vi "SetParam.vi"(7 "RS":bool, 8 "error in (no error)":errorcluster, 9 "Param to Set in":u16, 10 "Visa":refnum<visa-resource-name>) -> (0 "error out":errorcluster)   [LabVIEW 2017]
uses:
  <vilib>/Utility/miscctls.llb/LVMinMaxIncTypeDef.ctl
panel:
  out "RS Out":string
  out "Horizontal Progress Bar":i32(slide) min=0 max=50 scale=0.0..50.0
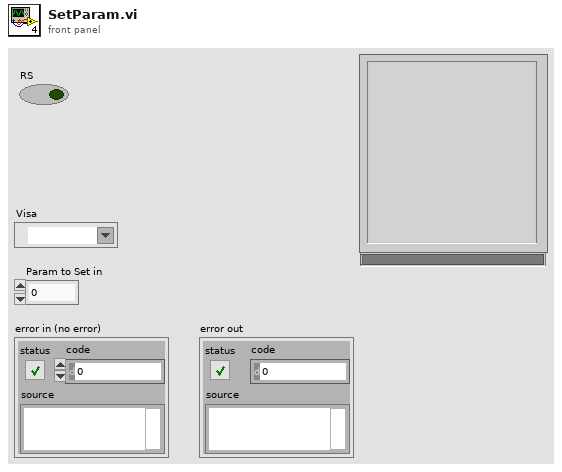
[diagram p1: front panel]
types:
  T1 = typedef "LVMinMaxIncTypeDef.ctl" = cluster{"Minimum":dbl, "Maximum":dbl, "Increment":dbl}
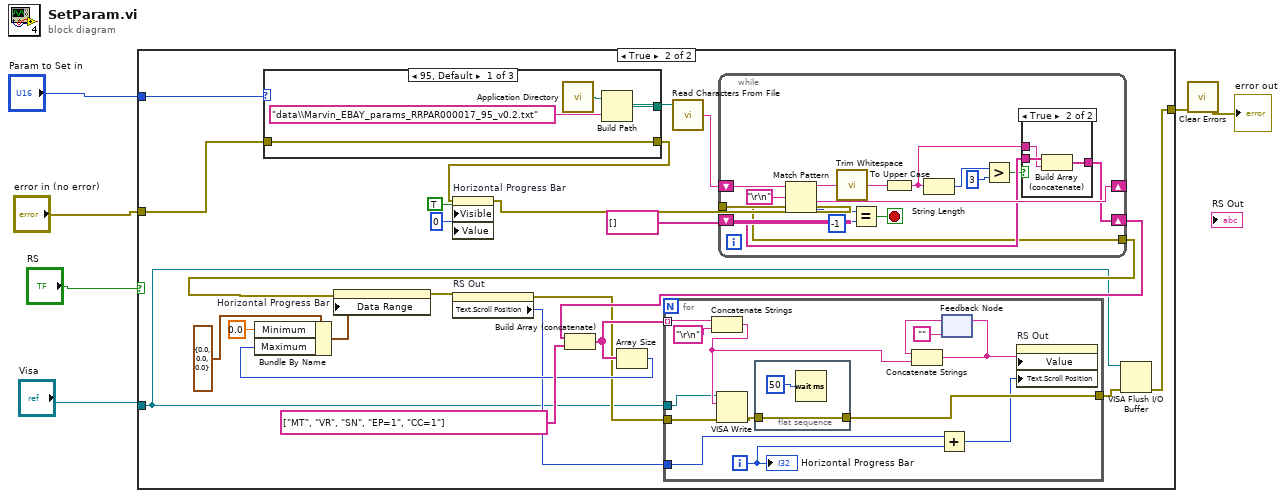
[diagram p0: block diagram]
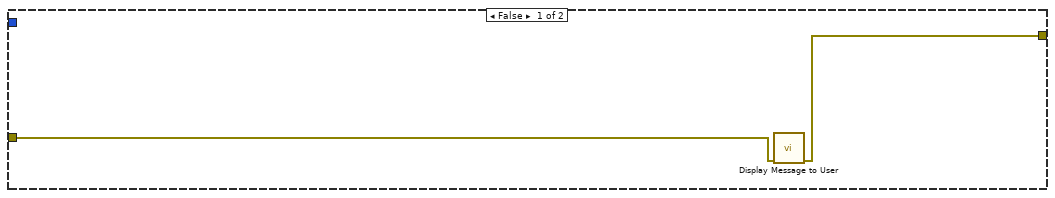
[diagram p2: hidden frame]
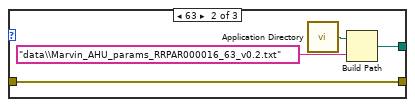
[diagram p4: hidden frame]
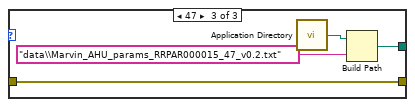
[diagram p5: hidden frame]
diagram:
  n1 = case shown="True" "RS" {
    tunnel: "error in (no error)" -> [w8 w18]
    tunnel: [w7 w15] -> w4
    tunnel: "Visa" -> [_ w10]
    tunnel: "Param to Set in" -> [_ w9]
    frame False {
      n2 = call "Display Message to User"("error in (no error)"=w8) -> ("error out"=w7:errorcluster)  [unwired: 9 in, 1 out]
    }
    frame True {
      n3 = case shown="95, Default" w9 {
        tunnel: [w67 w71 w75] -> w29
        tunnel: w18 -> [w66 w70 w74]
        tunnel: [w66 w70 w74] -> w21
        frame 95, Default {
          n4 = call <vilib>:"Application Directory.vi"() -> ("Application Directory"=w69:path)
          n5 = Build Path(base path=w69, name or relative path="data\\Marvin_EBAY_params_RRPAR000017_95_v0.2.txt") -> (appended path=w67:path)
        }
        frame 63 {
          n6 = call <vilib>:"Application Directory.vi"() -> ("Application Directory"=w73:path)
          n7 = Build Path(base path=w73, name or relative path="data\\Marvin_AHU_params_RRPAR000016_63_v0.2.txt") -> (appended path=w71:path)
        }
        frame 47 {
          n8 = call <vilib>:"Application Directory.vi"() -> ("Application Directory"=w77:path)
          n9 = Build Path(base path=w77, name or relative path="data\\Marvin_AHU_params_RRPAR000015_47_v0.2.txt") -> (appended path=w75:path)
        }
      }
      n10 = property on="Horizontal Progress Bar" class="Slide (strict)"(error in=w21, "Visible"=TRUE, "Value"=u8 0 ("Horizontal Progress Bar")) -> (error out=w17:errorcluster)  [unwired: 1 in, 1 out]
      n11 = call <vilib>:"Read Characters From File.vi"("file path (dialog if empty)"=w29) -> ("character string"=w30:string)  [unwired: 5 in, 3 out]
      n12 = while {
        shift-right: [w58] -> _
        shift-left: w30 -> [w59]
        shift-right: [w54] -> w19
        shift-left: string[] [] -> [w55]
        tunnel: w17 -> [w47]
        tunnel: [w47] -> w11
        stop <- w60 stop-if-true
        n13 = Match Pattern(string=w59, regular expression="\r\n") -> (before substring=w56:string, after substring=w58:string, offset past match=w57:i32)  [unwired: 1 in, 1 out]
        n14 = call <vilib>:"Trim Whitespace.vi"("string"=w56) -> ("trimmed string"=w53:string)  [unwired: 1 in]
        n15 = Equal?(x=w57, y=-1) -> (x = y?=w60:bool)
        n16 = To Upper Case(1:w53) -> (0:w51:string)
        n17 = String Length(string=w51) -> (length=w50:i32)
        n18 = Greater?(x=w50, y=3) -> (0:w48:bool)
        n19 = case shown="True" w48 {
          tunnel: w55 -> [w62 w65]
          tunnel: [w62 w64] -> w54
          tunnel: w51 -> [_ w63]
          frame False {
          }
          frame True {
            n20 = Build Array (concatenate)(w65, w63) -> (w64:string[])
          }
        }
      }
      n21 = Build Array (concatenate)(w19, string[] ["MT", "VR", "SN", "EP=1", "CC=1"] ("array")) -> (w25:string[])
      n22 = Array Size(array=w25) -> (size(s)=w20:i32)
      n23 = Bundle By Name(cluster=T1 {"Minimum"=0.0, "Maximum"=0.0, "Increment"=0.0} ("Data Entry Limits"), "Minimum"=0.0, "Maximum"=w20) -> (w23:T1)
      n24 = property on="Horizontal Progress Bar" class="Slide (strict)"(error in=w11, "Data Range"=w23) -> (error out=w14:errorcluster)  [unwired: 1 in, 1 out]
      n25 = property on="RS Out" class="Str"(error in=w14) -> (error out=w13:errorcluster, "Text.Scroll Position"=w12:u32)  [unwired: 1 in, 1 out]
      n26 = for {
        tunnel: w25 -> [w39] mode=indexing
        tunnel: w13 -> [w44]
        tunnel: [w36] -> w16
        tunnel: w12 -> [w35]
        tunnel: w10 -> [w32]
        i -> [w34]
        n27 = Concatenate Strings(w39, "\r\n" ("string")) -> (w37:string)
        n28 = VISA Write(VISA resource name=w32, write buffer=w37, error in (no error)=w44) -> (error out=w43:errorcluster)  [unwired: 2 out]
        n29 = flat-sequence {
          tunnel: w43 -> [w45]
          tunnel: [w45] -> w36
          frame #0 {
            n30 = Wait (ms)(milliseconds to wait=u32 50) -> ()  [unwired: 1 out]
          }
        }
        n31 = Add(x=w35, y=w34) -> (x+y=w33:u32)
        n32 = feedback #1("") -> (w41:string)
        n33 = Concatenate Strings(w41, w37) -> (w42:string)
        n34 = feedback-in #1(w42) -> ()
        n35 = property on="RS Out" class="Str"("Value"=w42, "Text.Scroll Position"=w33) -> ()  [unwired: 2 in, 2 out]
        "Horizontal Progress Bar" <- w34
      }
      n36 = VISA Flush I/O Buffer(VISA resource name=w10, error in (no error)=w16) -> (error out=w15:errorcluster)  [unwired: 1 in, 1 out]
    }
  }
  n37 = call <vilib>:"Clear Errors.vi"("error in (no error)"=w4) -> ("error out"=→"error out":errorcluster)  [unwired: 5 in, 1 out]
